vi "TinyPackets.vi"(2 "Max Size":i32=500, 3 "Translate":enum16{"None", "Tiny", "URAPI"}(ring), 4 "URAPI Script":T1={"Script"="count0=0\n//while0 forever\nforever:\ncount0=count0+1\nD!0=count0\ncount0+=1\ngoto forever\n", "Whiles"=[], "Ifs"=[], "Supress Err"=TRUE, "Errors"=""}) -> (1 "Script Packets":string[](array[string]))   [LabVIEW 2012]
uses:
  <userlib>/botspeak/VIs/Direct/URAPI_Control.ctl
  <userlib>/botspeak/VIs/SubVIs/BotSpeak_Globals.vi
panel:
  out "script":string="SET count0,0\n\nADD count0,1\nDIO 0,count0\nADD count0,1\ngoto 2\n"
  out "# chars":i32=28
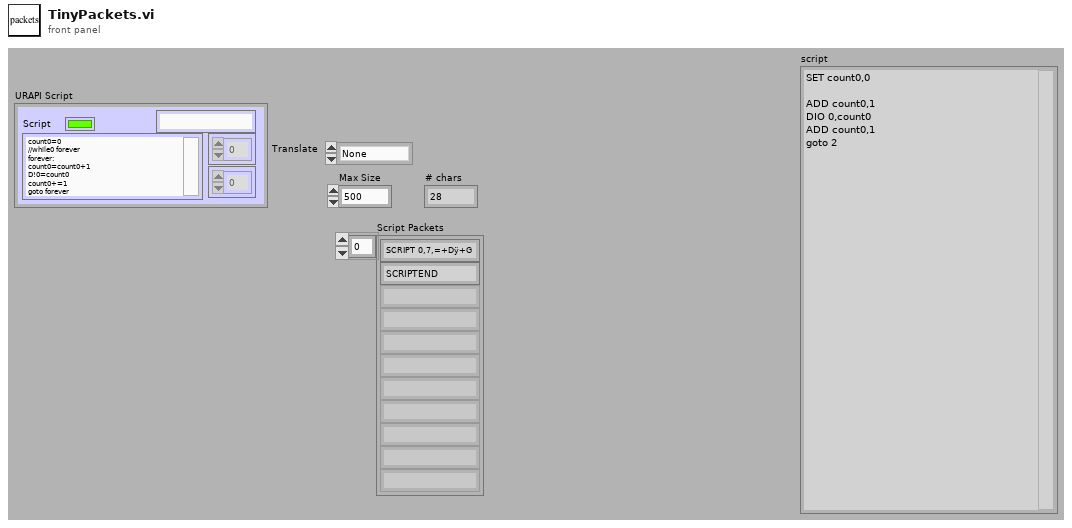
[diagram p1: front panel]
types:
  T1 = typedef "URAPI_Control.ctl" = cluster{"Script":string, "Whiles":u8[], "Ifs":u8[], "Supress Err":bool, "Errors":string}
  T2 = cluster{"Sent":string, "reply":string, "reply 2":string}[]
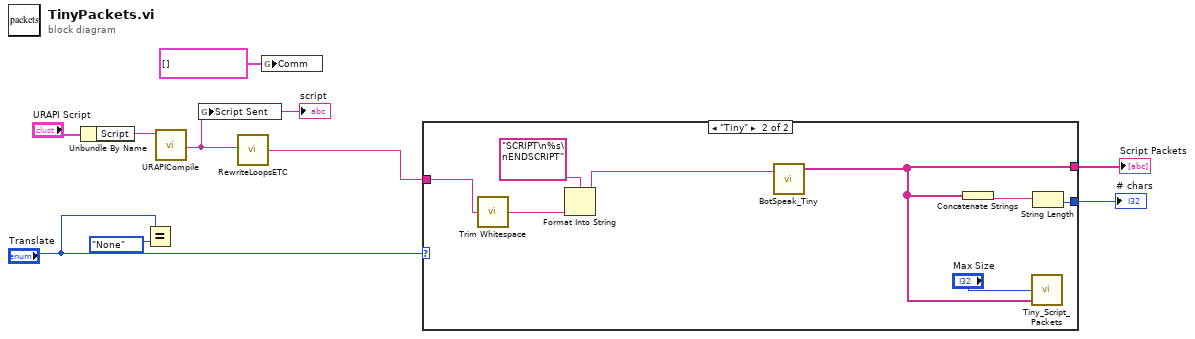
[diagram p0: block diagram]
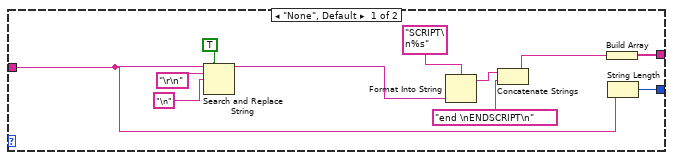
[diagram p2: hidden frame]
diagram:
  n1 = Unbundle By Name("URAPI Script") -> ("Script"=w6:string)
  n2 = Equal?(x="Translate", y=enum16{"None", "Tiny", "URAPI"}."None") -> ()  [unwired: 1 out]
  n3 = call <userlib>:"URAPICompile.vi"("Script"=w6) -> ("trimmed script"=w2:string)  [unwired: 1 in]
  "script" <- w2
  n4 = global write "BotSpeak_Globals.vi" "Script Sent"(w2) -> ()
  n5 = call <userlib>:"RewriteLoopsETC.vi"("URAPI in"=w2) -> ("URAPI out"=w1:string)  [unwired: 1 in]
  n6 = global write "BotSpeak_Globals.vi" "Comm"(T2 [] ("Comm")) -> ()
  n7 = case shown="\"Tiny\"" "Translate" {
    tunnel: [w19 w24] -> w8
    tunnel: [w20 w22] -> w7
    tunnel: w1 -> [w10 w26]
    frame "None", Default {
      n8 = Search and Replace String(replace all?=TRUE ("replace all? (F)"), input string=w10, search string="\r\n", replace string="\n" ("search string")) -> (result string=w15:string)  [unwired: 4 in, 3 out]
      n9 = Format Into String(format string="SCRIPT\n%s" ("command"), w15) -> (resulting string=w13:string)  [unwired: 2 in, 1 out]
      n10 = Concatenate Strings(w13, "end \nENDSCRIPT\n" ("search string")) -> (w12:string)
      n11 = Build Array(w12) -> (w19:string[])
      n12 = String Length(string=w10) -> (length=w20:i32)
    }
    frame "Tiny" {
      n13 = call <vilib>:"Trim Whitespace.vi"("string"=w26) -> ("trimmed string"=w25:string)  [unwired: 1 in]
      n14 = Format Into String(format string="SCRIPT\n%s\nENDSCRIPT" ("command"), w25) -> (resulting string=w27:string)  [unwired: 2 in, 1 out]
      n15 = call <userlib>:"BotSpeak_Tiny.vi"("URAPI"=w27) -> ("Tiny Lines"=w24:string[])  [unwired: 1 in, 2 out]
      n16 = Concatenate Strings(w24) -> (w23:string)
      n17 = call <userlib>:"Tiny_Script_Packets.vi"("Lines in"=w24, "Max Size"="Max Size") -> ()  [unwired: 1 in, 2 out]
      n18 = String Length(string=w23) -> (length=w22:i32)
    }
  }
  "Script Packets" <- w8
  "# chars" <- w7
